vi "Apply Style.vi"(8 "error in (no error)":errorcluster, 10 "Headers.Style":refnum<class "Style.lvclass">, 11 "xwpfParagraph in":refnum<class "xwpfParagraph.lvclass">) -> (0 "error out":errorcluster, 3 "xwpfParagraph out":refnum<class "xwpfParagraph.lvclass">)   [LabVIEW 2017, in "Word_Specific.lvlib" / "xwpfParagraph.lvclass"]
uses:
  xwpfParagraph.lvclass
  Styles/Style/Style.lvclass
  xwpfParagraph.lvclass/xwpfParagraph.ctl
  xwpfRun/xwpfRun.lvclass/xwpfRun.ctl
  xwpfRun/Set Style.vi
  Get Runs.vi
  xwpfRun/xwpfRun.lvclass
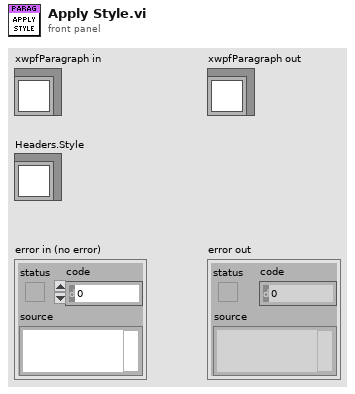
[diagram p1: front panel]
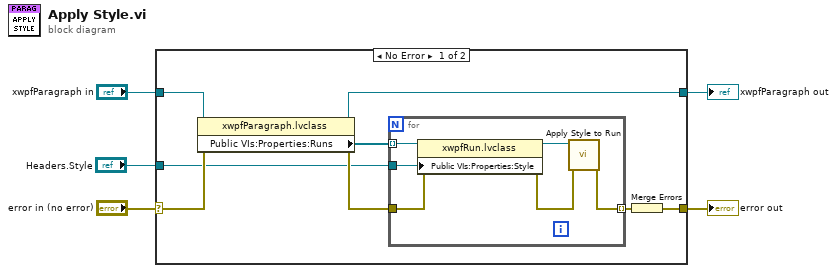
[diagram p0: block diagram]
diagram:
  n1 = case shown="No Error" "error in (no error)" {
    selector: "error in (no error)" -> [w8 w21]
    tunnel: [w7 w21] -> w4
    tunnel: [w12 w20] -> w2
    tunnel: "xwpfParagraph in" -> [w13 w20]
    tunnel: "Headers.Style" -> [w6 _]
    frame No Error {
      n2 = property class="xwpfParagraph.lvclass"(reference=w13, error in=w8) -> (reference out=w12:refnum<class "xwpfParagraph.lvclass">, error out=w10:errorcluster, "Public VIs:Properties:Runs"=w11:refnum<class "xwpfRun.lvclass">[])
      n3 = for {
        tunnel: w11 -> [w19] mode=indexing
        tunnel: [w18] -> w9 mode=indexing
        tunnel: w10 -> [w16]
        tunnel: w6 -> [w14]
        n4 = property class="xwpfRun.lvclass"(reference=w19, error in=w16, "Public VIs:Properties:Style"=w14) -> (reference out=w17:refnum<class "xwpfRun.lvclass">, error out=w15:errorcluster)
        n5 = call-dynamic "Apply Style to Run.vi"("error in (no error)"=w15, "xwpfRun in"=w17) -> ("error out"=w18:errorcluster)  [unwired: 8 in, 1 out]
      }
      n6 = Merge Errors(w9) -> (w7:errorcluster)
    }
    frame Error {
    }
  }
  "error out" <- w4
  "xwpfParagraph out" <- w2
